vi "Write Filter Shortcut Menu Activation Event.vi"(6 "Filter Shortcut Menu Activation Event":refnum<notifier>, 11 "Handle Activate Menu On Tree Item Msg in":refnum<class "Handle Activate Menu On Tree Item Msg.lvclass">) -> (3 "Handle Activate Menu On Tree Item Msg out":refnum<class "Handle Activate Menu On Tree Item Msg.lvclass">)   [LabVIEW 2017, in "File Explorer.lvlib" / "Handle Activate Menu On Tree Item Msg.lvclass"]
uses:
  <vilib>/gpm_packages/@cs/file-explorer-extension/Source/File Explorer/File Explorer Messages/Handle Activate Menu On Tree Item Msg/Handle Activate Menu On Tree Item Msg.lvclass
  <vilib>/gpm_packages/@cs/file-explorer-extension/Source/File Explorer/File Explorer Messages/Handle Activate Menu On Tree Item Msg/Handle Activate Menu On Tree Item Msg.lvclass/Handle Activate Menu On Tree Item Msg.ctl
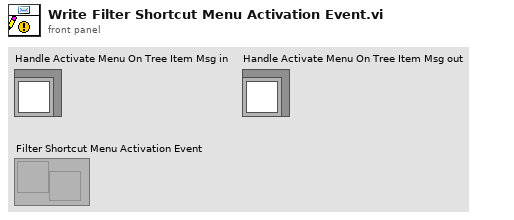
[diagram p1: front panel]
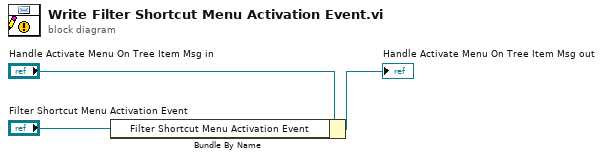
[diagram p0: block diagram]
diagram:
  n1 = Bundle By Name(cluster="Handle Activate Menu On Tree Item Msg in", "Filter Shortcut Menu Activation Event"="Filter Shortcut Menu Activation Event") -> (→"Handle Activate Menu On Tree Item Msg out":refnum<class "Handle Activate Menu On Tree Item Msg.lvclass">)
